vi "test 14- ChainModeCallsChainMode.vi"(8 "error in (no error)":errorcluster, 11 "TestCase in":refnum<class "testcase-SyncMessage.lvclass">) -> (0 "error out":errorcluster, 3 "TestCase out":refnum<class "testcase-SyncMessage.lvclass">)   [LabVIEW 2017, in "testcase-SyncMessage.lvclass"]
uses:
  testcase-SyncMessage.lvclass
  <vilib>/addons/_JKI Toolkits/VI Tester/TestCase.llb/TestCase.lvclass
  src/user.lib/_NEVSTOP/Communicable State Machine(CSM)/Communicable State Machine.lvlib
  C:/Program Files (x86)/National Instruments/LabVIEW 2017/vi.lib/addons/_JKI Toolkits/VI Tester/TestCase.llb/TestCase.lvclass
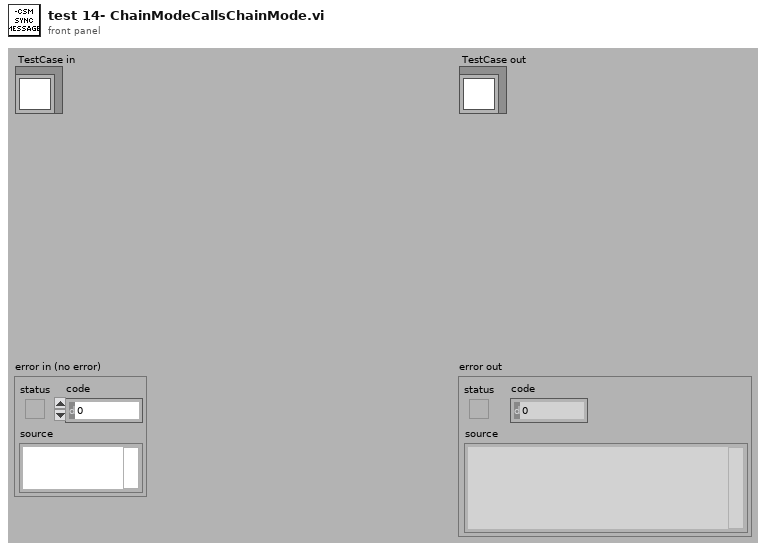
[diagram p1: front panel]
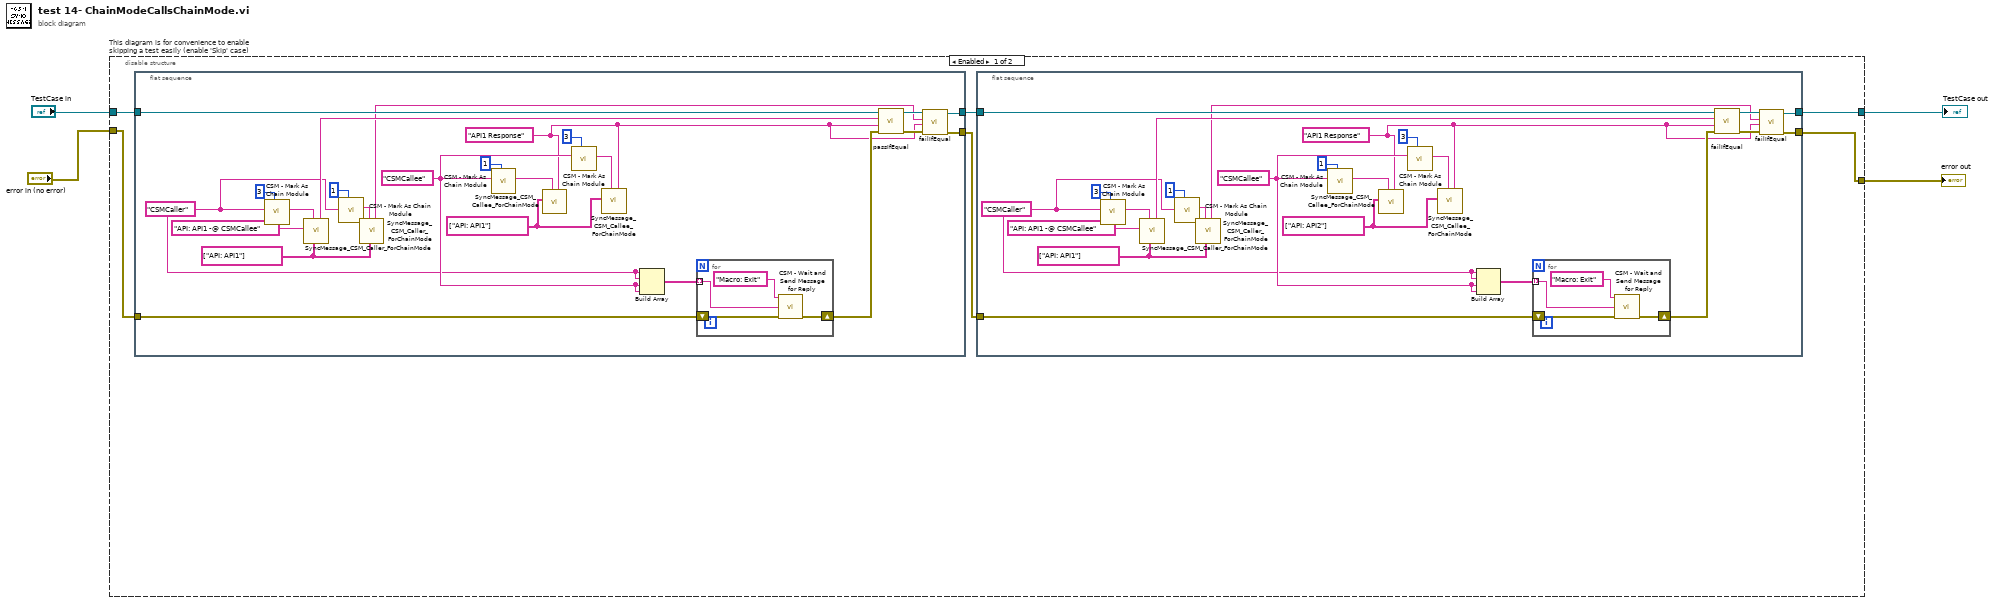
[diagram p0: block diagram]
diagram:
  n1 = disable-structure "This diagram is for convenience to enable skipping a test easily (enable 'Skip' case)" shown="Enabled" {
    disable-tunnel: "TestCase in" -> [w10 w70]
    disable-tunnel: [w6 w68] -> w2
    disable-tunnel: [w5 w69] -> w1
    disable-tunnel: "error in (no error)" -> [w9 w67]
    frame Enabled {
      n2 = flat-sequence {
        tunnel: w10 -> [w62]
        tunnel: [w42] -> w8
        tunnel: w9 -> [w54]
        tunnel: [w39] -> w7
        frame #0 {
          w48 = string[] ["API: API1"] ("Allowed Messages (Empty for All)")
          w57 = string[] ["API: API1"] ("Allowed Messages (Empty for All)")
          w51 = "CSMCallee" ("CSMCallee")
          w45 = "CSMCaller" ("CSMCaller")
          w40 = "API1 Response" ("API response in")
          n3 = call "CSM - Mark As Chain Module.vi"("Order"=3, "CSM Name"=w45) -> ("CSM Name (Marked As Chain)"=w52:string)  [unwired: 8 in]
          n4 = call "SyncMessage_CSM_Caller_ForChainMode.vi"("Allowed Messages (Empty for All)"=w48, "Name (\"\" to Use UUID)"=w52, "Intermodule Message in"="API: API1 -@ CSMCallee") -> ("API received Response out"=w49:string)  [unwired: 8 in]
          n5 = call "CSM - Mark As Chain Module.vi"("Order"=1, "CSM Name"=w45) -> ("CSM Name (Marked As Chain)"=w46:string)  [unwired: 8 in]
          n6 = call "SyncMessage_CSM_Caller_ForChainMode.vi"("Allowed Messages (Empty for All)"=w48, "Name (\"\" to Use UUID)"=w46) -> ("API received Response out"=w41:string)  [unwired: 9 in]
          n7 = call "CSM - Mark As Chain Module.vi"("Order"=1, "CSM Name"=w51) -> ("CSM Name (Marked As Chain)"=w58:string)  [unwired: 8 in]
          n8 = call "SyncMessage_CSM_Callee_ForChainMode.vi"("API response in"=w40, "Name (\"\" to Use UUID)"=w58, "Allowed Messages (Empty for All)"=w57) -> ()  [unwired: 9 in]
          n9 = call "CSM - Mark As Chain Module.vi"("Order"=3, "CSM Name"=w51) -> ("CSM Name (Marked As Chain)"=w55:string)  [unwired: 8 in]
          n10 = call "SyncMessage_CSM_Callee_ForChainMode.vi"("API response in"=w40, "Name (\"\" to Use UUID)"=w55, "Allowed Messages (Empty for All)"=w57) -> ()  [unwired: 9 in]
          n11 = Build Array(w45, w45, w51, w51) -> (w61:string[])
          n12 = for {
            shift-right: [w64] -> w60
            shift-left: w54 -> [w65]
            tunnel: w61 -> [w63] mode=indexing
            n13 = call "CSM - Wait and Send Message for Reply.vi"("State"="Macro: Exit", "Target Module"=w63, "Error In (No Error)"=w65) -> ("error out"=w64:errorcluster)  [unwired: 10 in, 2 out]
          }
          n14 = call-dynamic "passIfEqual.vi"("error in (no error)"=w60, "y"=w40, "x"=w49, "TestCase in"=w62) -> ("error out"=w44:errorcluster, "TestCase out"=w43:refnum<class "testcase-SyncMessage.lvclass">)  [unwired: 6 in]
          n15 = call-dynamic "failIfEqual.vi"("error in (no error)"=w44, "y"=w40, "x"=w41, "TestCase in"=w43) -> ("error out"=w39:errorcluster, "TestCase out"=w42:refnum<class "testcase-SyncMessage.lvclass">)  [unwired: 6 in]
        }
      }
      n16 = flat-sequence {
        tunnel: w8 -> [w34]
        tunnel: [w14] -> w6
        tunnel: w7 -> [w26]
        tunnel: [w11] -> w5
        frame #0 {
          w20 = string[] ["API: API1"] ("Allowed Messages (Empty for All)")
          w29 = string[] ["API: API2"] ("Allowed Messages (Empty for All)")
          w23 = "CSMCallee" ("CSMCallee")
          w17 = "CSMCaller" ("CSMCaller")
          w12 = "API1 Response" ("API response in")
          n17 = call "CSM - Mark As Chain Module.vi"("Order"=3, "CSM Name"=w17) -> ("CSM Name (Marked As Chain)"=w24:string)  [unwired: 8 in]
          n18 = call "SyncMessage_CSM_Caller_ForChainMode.vi"("Allowed Messages (Empty for All)"=w20, "Name (\"\" to Use UUID)"=w24, "Intermodule Message in"="API: API1 -@ CSMCallee") -> ("API received Response out"=w21:string)  [unwired: 8 in]
          n19 = call "CSM - Mark As Chain Module.vi"("Order"=1, "CSM Name"=w17) -> ("CSM Name (Marked As Chain)"=w18:string)  [unwired: 8 in]
          n20 = call "SyncMessage_CSM_Caller_ForChainMode.vi"("Allowed Messages (Empty for All)"=w20, "Name (\"\" to Use UUID)"=w18) -> ("API received Response out"=w13:string)  [unwired: 9 in]
          n21 = call "CSM - Mark As Chain Module.vi"("Order"=1, "CSM Name"=w23) -> ("CSM Name (Marked As Chain)"=w30:string)  [unwired: 8 in]
          n22 = call "SyncMessage_CSM_Callee_ForChainMode.vi"("API response in"=w12, "Name (\"\" to Use UUID)"=w30, "Allowed Messages (Empty for All)"=w29) -> ()  [unwired: 9 in]
          n23 = call "CSM - Mark As Chain Module.vi"("Order"=3, "CSM Name"=w23) -> ("CSM Name (Marked As Chain)"=w27:string)  [unwired: 8 in]
          n24 = call "SyncMessage_CSM_Callee_ForChainMode.vi"("API response in"=w12, "Name (\"\" to Use UUID)"=w27, "Allowed Messages (Empty for All)"=w29) -> ()  [unwired: 9 in]
          n25 = Build Array(w17, w17, w23, w23) -> (w33:string[])
          n26 = for {
            shift-right: [w36] -> w32
            shift-left: w26 -> [w37]
            tunnel: w33 -> [w35] mode=indexing
            n27 = call "CSM - Wait and Send Message for Reply.vi"("State"="Macro: Exit", "Target Module"=w35, "Error In (No Error)"=w37) -> ("error out"=w36:errorcluster)  [unwired: 10 in, 2 out]
          }
          n28 = call-dynamic "failIfEqual.vi"("error in (no error)"=w32, "y"=w12, "x"=w21, "TestCase in"=w34) -> ("error out"=w16:errorcluster, "TestCase out"=w15:refnum<class "testcase-SyncMessage.lvclass">)  [unwired: 6 in]
          n29 = call-dynamic "failIfEqual.vi"("error in (no error)"=w16, "y"=w12, "x"=w13, "TestCase in"=w15) -> ("error out"=w11:errorcluster, "TestCase out"=w14:refnum<class "testcase-SyncMessage.lvclass">)  [unwired: 6 in]
        }
      }
    }
    frame Disabled {
      # "skip test result while test is under development"
      n30 = call <vilib>:"skip.vi"("error in (no error)"=w67, "TestCase in"=w70) -> ("error out"=w69:errorcluster, "TestCase out"=w68:refnum<class "testcase-SyncMessage.lvclass">)  [unwired: 8 in]
    }
  }
  "error out" <- w1
  "TestCase out" <- w2
